vi "RP100.Get Level.vi"(8 "error in (no error)":errorcluster, 10 "Output Channel":T1, 11 "VISA resource name":refnum<visa-resource-name>) -> (0 "error out":errorcluster, 1 "Level (V)":dbl, 2 "Output Channel":T1, 3 "VISA Refnum out":refnum<visa-resource-name>)   [LabVIEW 2019, in "Inst.RP100.lvclass"]
uses:
  Inst.RP100.lvclass
  Typedefs/Channel--Num.ctl
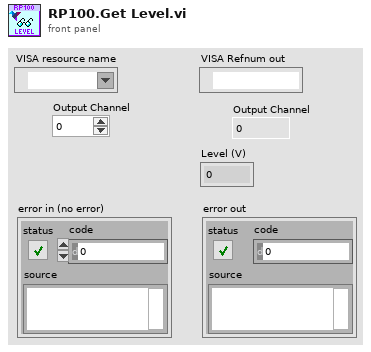
[diagram p1: front panel]
types:
  T1 = typedef "Inst.RP100.lvclass/Channel--Num.ctl" = i32
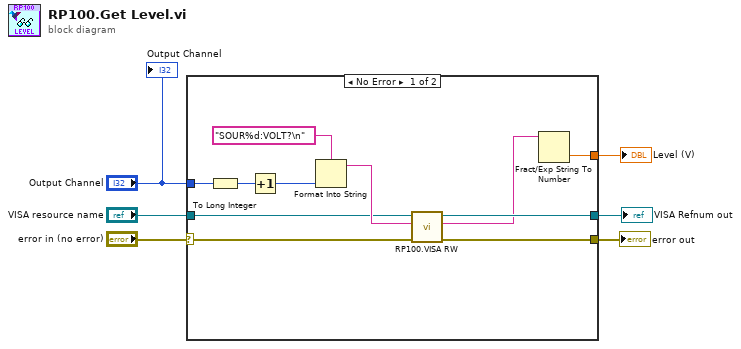
[diagram p0: block diagram]
diagram:
  n1 = case shown="No Error" "error in (no error)" {
    selector: "error in (no error)" -> [w14 w18]
    tunnel: "VISA resource name" -> [w12 w19]
    tunnel: "Output Channel" -> [w16 _]
    tunnel: [w17 _] -> w4
    tunnel: [w11 w19] -> w3
    tunnel: [w9 w18] -> w2
    frame No Error {
      n2 = To Long Integer(number=w16) -> (32bit integer=w8:T1)
      n3 = Increment(x=w8) -> (x+1=w7:T1)
      n4 = Format Into String(format string="SOUR%d:VOLT?\n", w7) -> (resulting string=w13:string)  [unwired: 2 in, 1 out]
      n5 = call "RP100.VISA RW.vi"("error in (no error)"=w14, "Write"=w13, "VISA Refnum in"=w12) -> ("error out"=w9:errorcluster, "Read"=w10:string, "VISA Refnum out"=w11:refnum<visa-resource-name>)  [unwired: 6 in]
      n6 = Fract/Exp String To Number(string=w10) -> (number=w17:dbl)  [unwired: 3 in, 1 out]
    }
    frame Error {
    }
  }
  "error out" <- w2
  "VISA Refnum out" <- w3
  "Level (V)" <- w4
  "Output Channel" <- "Output Channel"
